vi "Tools Bar Example.vi"() -> ()   [LabVIEW 2016]
panel:
  out "Image":T1(plugin-control)
  in  "stop":bool
  out "Image 2":T1(plugin-control)
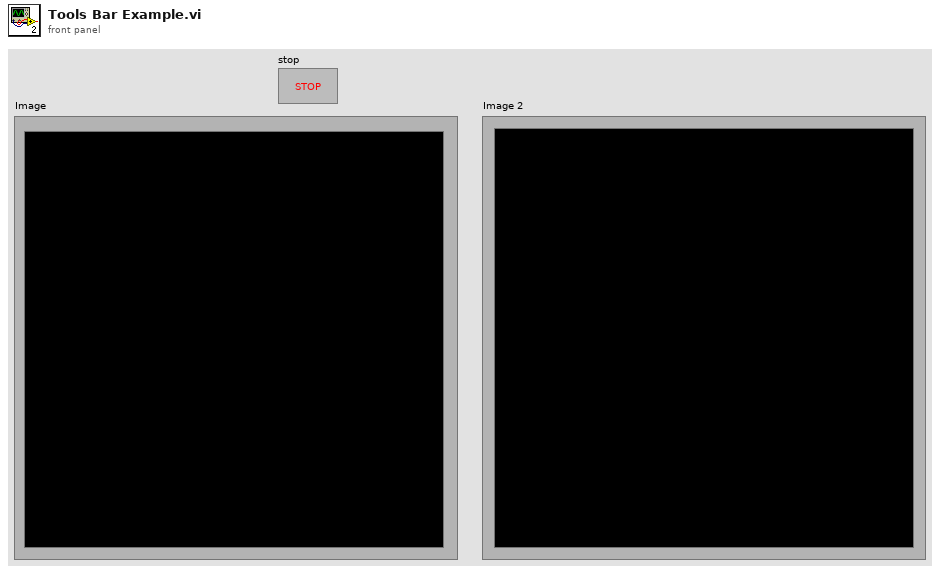
[diagram p1: front panel]
types:
  T1 = typedef "IMAQ Image.ctl" = refnum<image>
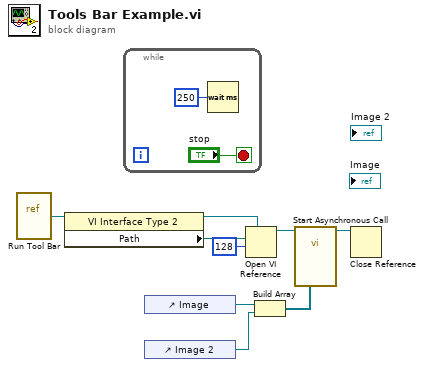
[diagram p0: block diagram]
diagram:
  n1 = vi-ref "Run Tool Bar.vi"() -> (w7:refnum<vi>)
  n2 = property class="VI Interface Type 2"(reference=w7) -> (reference out=w3:refnum<vi>, "Path"=w6:path)  [unwired: 1 in, 1 out]
  n3 = while {
    stop <- "stop" stop-if-true
    n4 = Wait (ms)(milliseconds to wait=u32 250) -> ()  [unwired: 1 out]
  }
  n5 = control-ref of="Image"() -> (w8:refnum<vi>)
  n6 = control-ref of="Image 2"() -> (w9:refnum<vi>)
  n7 = Open VI Reference(type specifier VI Refnum (for type only)=w3, vi path=w6, options=128) -> (vi reference=w2:refnum<vi>)  [unwired: 3 in, 1 out]
  n8 = Build Array(w8, w9) -> (w1:refnum<vi>[])
  n9 = call-by-ref "Start Asynchronous Call"(reference=w2, "IMAQ Display Refs"=w1) -> (reference out=w4:refnum<vi>)  [unwired: 16 in, 1 out]
  n10 = Close Reference(reference=w4) -> ()  [unwired: 1 in, 1 out]
